vi "LoadFromDisk.vi"(8 "Error In":errorcluster, 10 "FileName":string, 11 "reference in":refnum<class "RealImage.lvclass">) -> (0 "Error Out":errorcluster, 3 "reference out":refnum<class "RealImage.lvclass">)   [LabVIEW 2020, in "RealImage.lvclass"]
uses:
  RealImage.lvclass
  Console_class/Console.lvclass
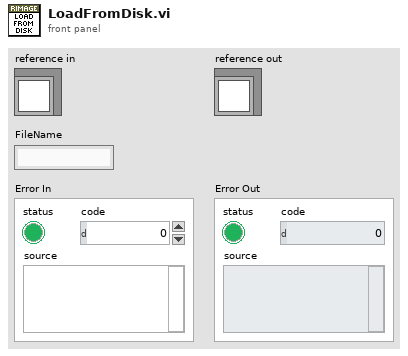
[diagram p1: front panel]
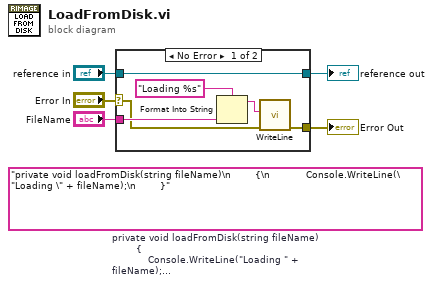
[diagram p0: block diagram]
diagram:
  (unwired) "private void loadFromDisk(string fileName)\n        {\n            Console.WriteLine(\"Loading \" + fileName);\n        }"  # private void loadFromDisk(string fileName)         {             Console.WriteLine("Loading " + fileName);         }
  n1 = case shown="No Error" "Error In" {
    selector: "Error In" -> [w7 w13]
    tunnel: [w6 w13] -> w4
    tunnel: [w11 w12] -> w2
    tunnel: "reference in" -> [w11 w12]
    tunnel: "FileName" -> [w9 _]
    frame No Error {
      n2 = Format Into String(format string="Loading %s", w9) -> (resulting string=w8:string)  [unwired: 2 in, 1 out]
      n3 = call "WriteLine.vi"("Error In"=w7, "ConsoleText"=w8) -> ("Error Out"=w6:errorcluster)  [unwired: 9 in]
    }
    frame Error {
    }
  }
  "Error Out" <- w4
  "reference out" <- w2
